vi "get_terminal_name_with_prefix.vi"(8 "error in (no error)":errorcluster, 10 "Local Terminal Name":string, 11 "task in":refnum<k21> caption="task/channels in") -> (0 "error out":errorcluster, 2 "Terminal Name with Device Prefix":tag, 3 "task out":refnum<k21>)   [LabVIEW 2010, in "ClockDL100201DAQmx.lvclass"]
doc: "This example takes in a DAQmx Task and a terminal and converts this to a terminal which includes the device prefix specified in the DAQmx Physical Channel Control.\n\nFor example: \nDAQmx Task in=Dev1/ctr1\nTerminal=InternalOutput\nDevice+Terminal=/Dev1/ctr1/InternalOutput"
uses:
  ClockDL100201DAQmx.lvclass
  Program Files/National Instruments/LabVIEW 2010/resource/objmgr/daqmx.rc
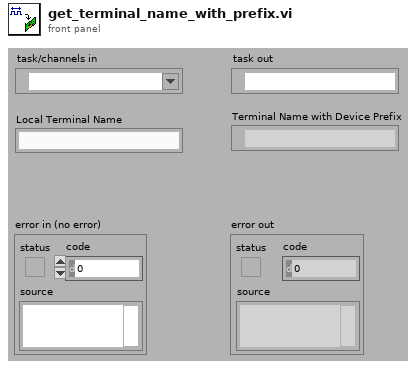
[diagram p1: front panel]
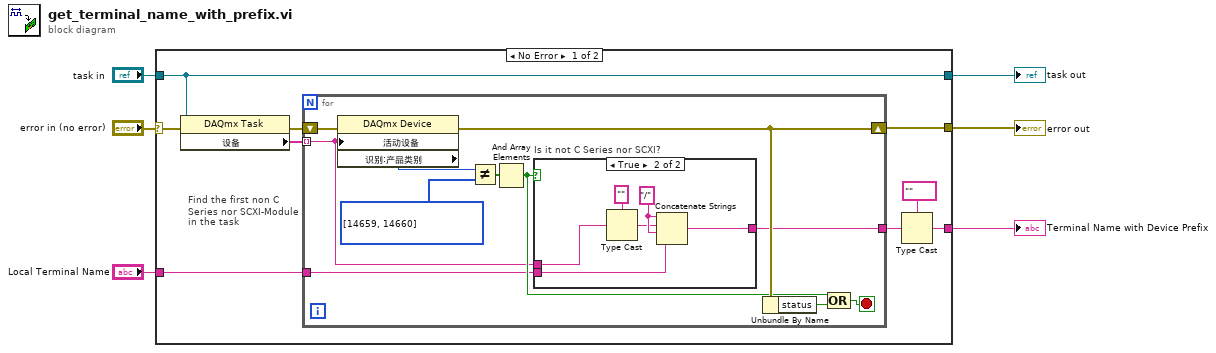
[diagram p0: block diagram]
diagram:
  n1 = case shown="No Error" "error in (no error)" {
    selector: "error in (no error)" -> [w12 w34]
    tunnel: "task in" -> [w8 w33]
    tunnel: [w14 w34] -> w5
    tunnel: [w11 _] -> w3
    tunnel: [w8 w33] -> w2
    tunnel: "Local Terminal Name" -> [w7 _]
    frame No Error {
      n2 = property class="DAQmx Task"(reference=w8, error in=w12) -> (error out=w15:errorcluster, "设备"=w13:tag[])  [unwired: 1 out]
      n3 = for "Find the first non C Series nor SCXI-Module in the task" {
        tunnel: w13 -> [w16] mode=indexing
        shift-right: [w22] -> w14
        shift-left: w15 -> [w23]
        tunnel: [w19] -> w10
        tunnel: w7 -> [w18]
        stop <- w17 stop-if-true
        w25 = i32[] [14659, 14660] items=["M Series DAQ"=14643, "E Series DAQ"=14642, "S Series DAQ"=14644, "B Series DAQ"=14662, "SC Series DAQ"=14645, "USB DAQ"=14646, "AO Series"=14647, "Digital I/O"=14648, "TIO Series"=14661, "Dynamic Signal Acquisition"=14649, "Switches"=14650, "C Series Chassis"=14658, "C Series Module"=14659, "SCXI Module"=14660, "Unknown"=12588]
        n4 = property class="DAQmx Device"(error in=w23, "活动设备"=w16) -> (error out=w22:errorcluster, "识别:产品类别"=w26:i32)  [unwired: 1 in, 1 out]
        n5 = Not Equal?(x=w26, y=w25) -> (x != y?=w24:bool[])
        n6 = And Array Elements(Boolean array=w24) -> (logical AND=w21:bool)
        n7 = case "Is it not C Series nor SCXI?" shown="True" w21 {
          tunnel: w16 -> [_ w29]
          tunnel: [_ w31] -> w19
          tunnel: w18 -> [_ w30]
          frame False {
            # "Module Case do nothing"
          }
          frame True {
            w32 = "/" ("string")
            n8 = Type Cast(type="", x=w29) -> (*(type *) &x=w28:string)
            n9 = Concatenate Strings(w32, w28, w32, w30) -> (w31:string)
          }
        }
        n10 = Unbundle By Name(w22) -> ("status"=w20:bool)
        n11 = Compound Arithmetic op=OR(w21, w20) -> (w17:bool)
      }
      n12 = Type Cast(type=tag "" ("Terminal Name with Device Prefix"), x=w10) -> (*(type *) &x=w11:tag)
    }
    frame Error {
    }
  }
  "error out" <- w5
  "Terminal Name with Device Prefix" <- w3
  "task out" <- w2
